vi "4461 Autophase.vi"(8 "error in (no error)":errorcluster, 10 "Results":T1, 11 "Lockin":refnum<class "Instrument.Lockin.lvclass">) -> (0 "error out":errorcluster, 3 "Lockin out":refnum<class "Instrument.Lockin.lvclass">)   [LabVIEW 2016, in "Instrument.Lockin.lvclass"]
uses:
  Instrument.Lockin.lvclass
  Typedefs/Results--Cluster.ctl
  Instrument.Lockin.lvclass/Instrument.Lockin.ctl
panel:
  in  "D":dbl=0.019999999999999997 format="%.2f"
  in  "I":dbl=0.6 format="%.2f"
  in  "P":dbl=0.5 format="%.2f"
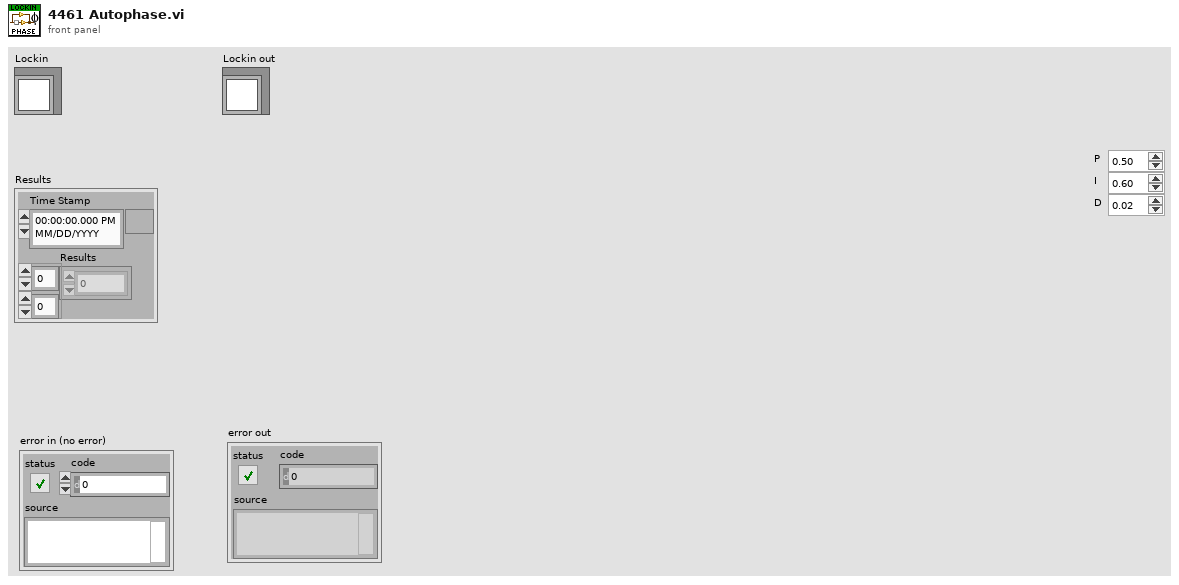
[diagram p1: front panel]
types:
  T1 = typedef "Instrument.Lockin.lvclass/Results--Cluster.ctl" = cluster{"Time Stamp":timestamp, "Results":dbl[][]}
  T2 = typedef "Instrument.Lockin.lvclass/REF_phi-array.ctl" = dbl[]
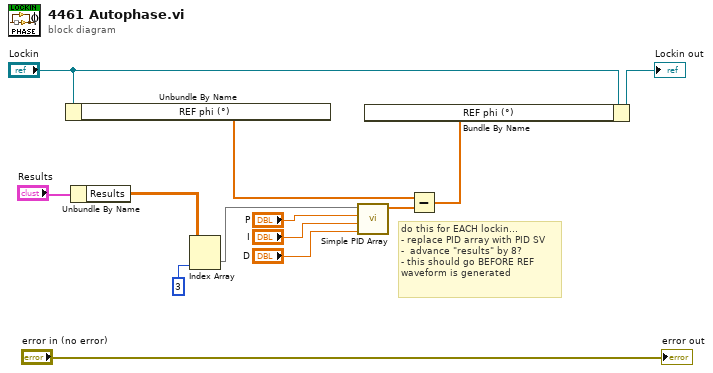
[diagram p0: block diagram]
diagram:
  # "do this for EACH lockin...\n- replace PID array with PID SV\n-  advance \"results\" by 8?\n- this should go BEFORE REF\nwaveform is generated"
  n1 = Unbundle By Name("Lockin") -> ("REF phi (°)"=w3:T2)
  n2 = Unbundle By Name("Results") -> ("Results"=w1:dbl[][])
  n3 = Index Array(array=w1, index (col)=3 ("index (row)")) -> (element=w8:dbl[])  [unwired: 1 in]
  n4 = call "Simple PID Array.vi"("D"="D", "I"="I", "P"="P", "process variable"=w8) -> ("output value"=w12:dbl[])  [unwired: 7 in]
  n5 = Subtract(x=w3, y=w12) -> (x-y=w6:T2)
  n6 = Bundle By Name(cluster="Lockin", "REF phi (°)"=w6) -> (→"Lockin out":refnum<class "Instrument.Lockin.lvclass">)
  "error out" <- "error in (no error)"
